vi "Get Tiles Info.vi"(8 "error in (no error)":errorcluster, 11 "Tiles Info Msg in":refnum<class "Tiles Info Msg.lvclass">) -> (0 "error out":errorcluster, 2 "Tiles Info":string[][](array[string]), 3 "Tiles Info Msg out":refnum<class "Tiles Info Msg.lvclass">)   [LabVIEW 2013, in "Project Model.lvlib" / "Tiles Info Msg.lvclass"]
uses:
  Tiles Info Msg.lvclass
  Tiles Info Msg.lvclass/Tiles Info Msg.ctl
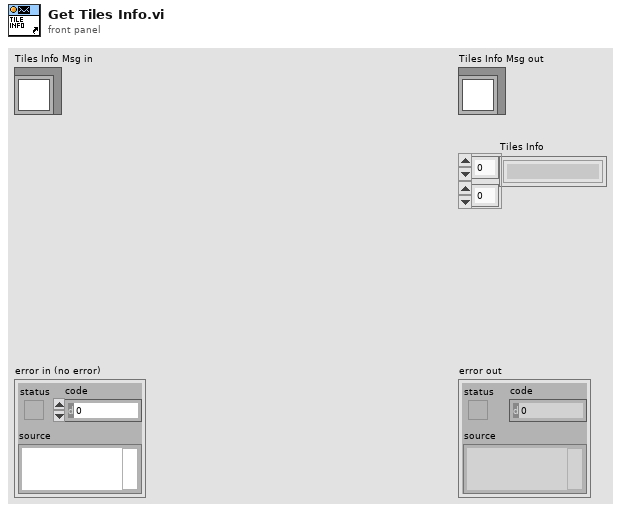
[diagram p1: front panel]
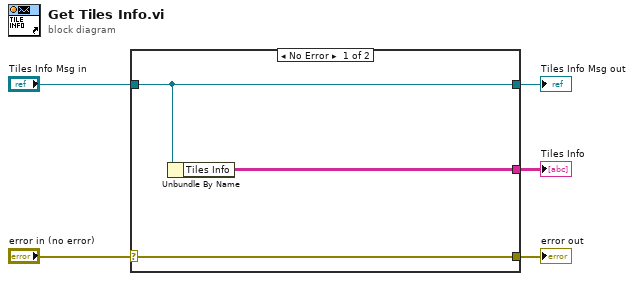
[diagram p0: block diagram]
diagram:
  n1 = case shown="No Error" "error in (no error)" {
    selector: "error in (no error)" -> [w8 w9]
    tunnel: [w8 w9] -> w4
    tunnel: [w7 w10] -> w2
    tunnel: "Tiles Info Msg in" -> [w7 w10]
    tunnel: [w6 _] -> w1
    frame No Error {
      n2 = Unbundle By Name(w7) -> ("Tiles Info"=w6:string[][])
    }
    frame Error {
    }
  }
  "error out" <- w4
  "Tiles Info Msg out" <- w2
  "Tiles Info" <- w1
